vi "Core Stream Controller.vi"(0 "input valid":bool, 1 "reset":bool, 5 "start trigger":bool, 7 "abort":bool, 9 "burst size":u32, 12 "samples per cycle":u32=1) -> (4 "write stream":bool, 6 "state":T1, 8 "samples processed":u32)   [LabVIEW 2015]
doc: "Controls whether the running state of the input/output streaming process is active or idle."
uses:
  Stream Control State.ctl
  Stream Control Parameters.ctl
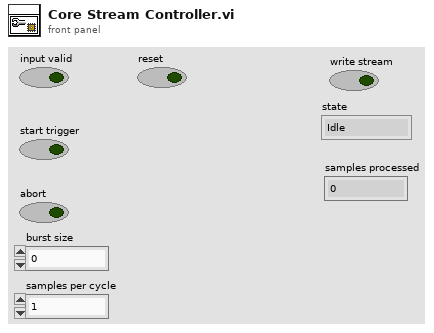
[diagram p1: front panel]
types:
  T1 = typedef "Stream Control State.ctl" = enum16{"Idle", "Active"}
  T2 = typedef "Stream Control Parameters.ctl" = cluster{"finite":bool, "samples remaining":u32, "state":T1, "samples processed":u32}
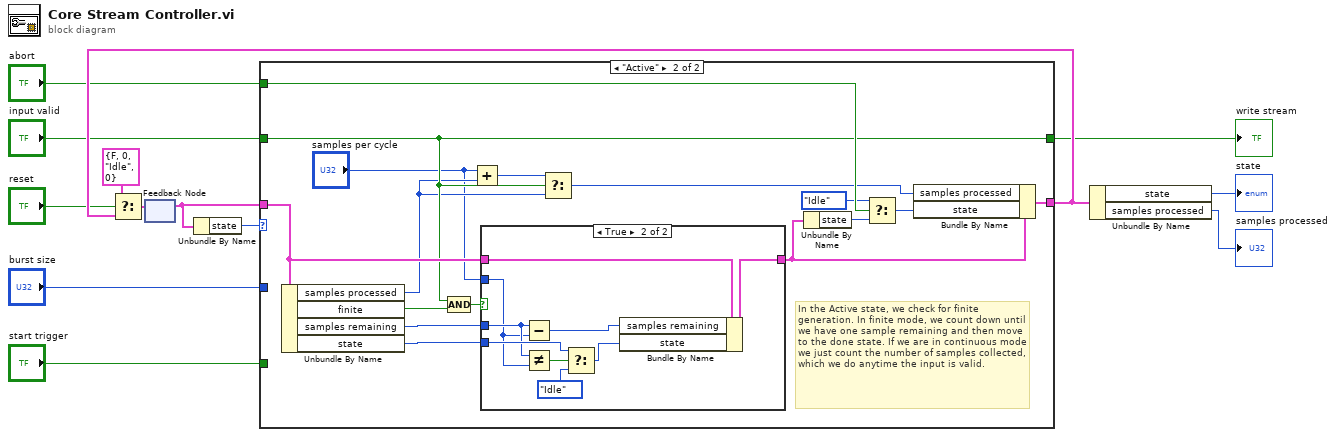
[diagram p0: block diagram]
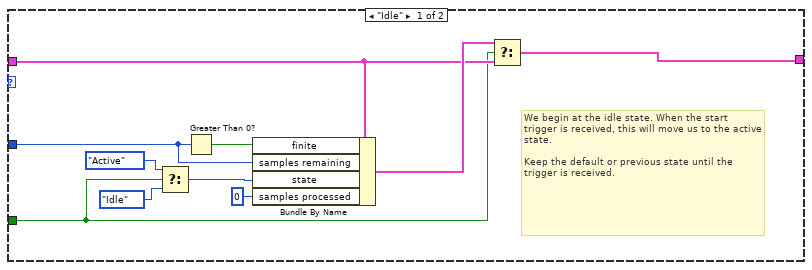
[diagram p2: hidden frame]
diagram:
  n1 = feedback #1() -> (w10:T2)  [unwired: 1 in]
  n2 = Unbundle By Name(w10) -> ("state"=w11:T1)
  n3 = case shown="\"Active\"" w11 {
    tunnel: "input valid" -> [_ w28]
    tunnel: w10 -> [w16 w39]
    tunnel: "burst size" -> [w22 _]
    tunnel: [w17 w31] -> w12
    tunnel: [_ w28] -> w2
    tunnel: "start trigger" -> [w15 _]
    tunnel: "abort" -> [_ w30]
    frame "Idle" {
      # "We begin at the idle state. When the start trigger is received, this will move us to the active state. \n\nKeep the default or previous state until the trigger is received."
      n4 = Select(t=Stream_Control_State."Active", s=w15, f=Stream_Control_State."Idle" ("t")) -> (s? t:f=w19:T1)
      n5 = Greater Than 0?(x=w22) -> (x > 0?=w23:bool)
      n6 = Bundle By Name(cluster=w16, "finite"=w23, "samples remaining"=w22, "state"=w19, "samples processed"=u32 0) -> (w18:T2)
      n7 = Select(t=w18, s=w15, f=w16) -> (s? t:f=w17:T2)
    }
    frame "Active" {
      # "In the Active state, we check for finite generation. In finite mode, we count down until we have one sample remaining and then move to the done state. If we are in continuous mode we just count the number of samples collected, which we do anytime the input is valid."
      n8 = Unbundle By Name(w39) -> ("samples processed"=w26:u32, "finite"=w37:bool, "samples remaining"=w38:u32, "state"=w35:T1)
      n9 = Compound Arithmetic op=AND(w28, w37) -> (w36:bool)
      n10 = Add(x="samples per cycle", y=w26) -> (x+y=w25:u32)
      n11 = case shown="True" w36 {
        tunnel: [w40 w49] -> w32
        tunnel: w39 -> [w40 w48]
        tunnel: w38 -> [_ w43]
        tunnel: w35 -> [_ w45]
        tunnel: "samples per cycle" -> [_ w41]
        frame False {
        }
        frame True {
          n12 = Subtract(x=w43, y=w41) -> (x-y=w42:u32)
          n13 = Not Equal?(x=w43, y=w41) -> (x != y?=w47:bool)
          n14 = Select(t=w45, s=w47, f=Stream_Control_State."Idle" ("state")) -> (s? t:f=w46:T1)
          n15 = Bundle By Name(cluster=w48, "samples remaining"=w42, "state"=w46) -> (w49:T2)
        }
      }
      n16 = Select(t=w25, s=w28, f=w26) -> (s? t:f=w27:u32)
      n17 = Unbundle By Name(w32) -> ("state"=w34:T1)
      n18 = Select(t=Stream_Control_State."Idle", s=w30, f=w34) -> (s? t:f=w33:T1)
      n19 = Bundle By Name(cluster=w32, "samples processed"=w27, "state"=w33) -> (w31:T2)
    }
  }
  "write stream" <- w2
  n20 = Select(t=T2 {"finite"=FALSE, "samples remaining"=0, "state"=enum."Idle", "samples processed"=0} ("Cluster"), s="reset", f=w12) -> (s? t:f=w9:T2)
  n21 = feedback-in #1(w9) -> ()
  n22 = Unbundle By Name(w12) -> ("state"=→"state":T1, "samples processed"=→"samples processed":u32)
